vi "Global_HW_Address_Assignments.vi"() -> ()   [LabVIEW 2017]
uses:
  <vilib>/Rock Robotics/WPI/Joystick/WPI_JoystickDeviceEnum.ctl
  <vilib>/Rock Robotics/SystemInterfaces/DIO/FPGA_DIOChannel.ctl
  Claw Testing/Systems/WCDrive2018/Cluster_WCDrive_SetupData.ctl
  <vilib>/Rock Robotics/SystemInterfaces/AI/FPGA_AIChannel.ctl
  <vilib>/Rock Robotics/WPI/Solenoid/WPI_SolenoidChannel.ctl
  _SHARE ALL/RoboRio Share All/SRX Share All/TypeDefs SRX/Cluster_SRX_OPEN Data.ctl
panel:
  in  "InTake Setup":T1
  in  "WC Shift":T2
  in  "Sonar Scaling Factor":dbl=0.0235
  in  "Sonar Average Bits":u8
  in  "Sonar Channel":T3=enum."AI 3"
  in  "HW SETUP_WC Drive":T4={"Left Master"=15, "Invert Left Master"=TRUE, "Left Slave"=11, "Invert Left Slave"=FALSE, "Right Master"=16, "Invert Right Master"=TRUE, "Right Slave"=10, "Invert Right Slave"=FALSE, "Invert Left Encoder"=FALSE, "Invert Right Encoder"=FALSE}
  in  "Motor ID":u8
  in  "DIO Channel":T5=enum."DIO 1"
  in  "Button Board":T6=enum."USB 1"
  in  "Joystick":T6
  out "Invert Climber Motor":bool
  in  "Climber Motor":u8=5
  # "#HW_Adress\nAssign Motor Addresses\nWhen Given\nAssign in Global_HW_Address_Assignment.vi"
  # "#HW_Assigments These globals are used to assign\nthe HW settings for the robot. HW state machines should\nuse these global variables to ease updates if any HW\nchanges have been made."
  # "Sonar"
  # "Controllers"
  # "Climber"
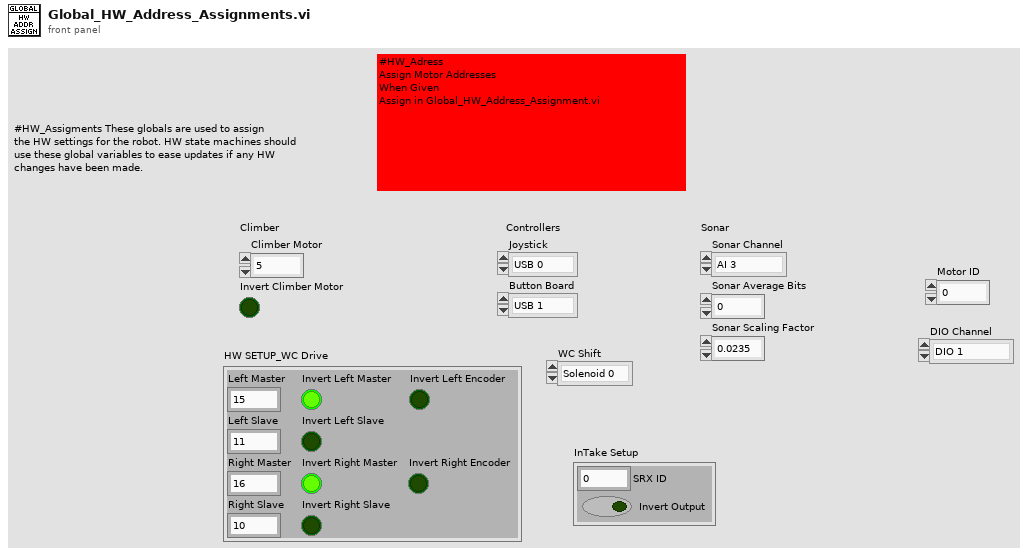
[diagram p1: front panel]
types:
  T1 = typedef "Cluster_SRX_OPEN Data.ctl" = cluster{"SRX ID":u8, "Invert Output":bool}
  T2 = typedef "WPI_SolenoidChannel.ctl" = enum8{"Solenoid 0", "Solenoid 1", "Solenoid 2", "Solenoid 3", "Solenoid 4", "Solenoid 5", "Solenoid 6", "Solenoid 7", "Invalid"}
  T3 = typedef "FPGA_AIChannel.ctl" = enum8{"AI 0", "AI 1", "AI 2", "AI 3", "AI MXP 0", "AI MXP 1", "AI MXP 2", "AI MXP 3", "Invalid"}
  T4 = typedef "Cluster_WCDrive_SetupData.ctl" = cluster{"Left Master":u8, "Invert Left Master":bool, "Left Slave":u8, "Invert Left Slave":bool, "Right Master":u8, "Invert Right Master":bool, "Right Slave":u8, "Invert Right Slave":bool, "Invert Left Encoder":bool, "Invert Right Encoder":bool}
  T5 = typedef "FPGA_DIOChannel.ctl" = enum8{"DIO 0", "DIO 1", "DIO 2", "DIO 3", "DIO 4", "DIO 5", "DIO 6", "DIO 7", "DIO 8", "DIO 9", "DIO MXP 0", "DIO MXP 1", "DIO MXP 2", "DIO MXP 3", "DIO MXP 4", "DIO MXP 5", "DIO MXP 6", "DIO MXP 7", "DIO MXP 8", "DIO MXP 9", "DIO MXP 10", "DIO MXP 11", "DIO MXP 12", "DIO MXP 13", "DIO MXP 14", "DIO MXP 15", "SPI Port CS1", "SPI Port CS2", "SPI Port CS3", "SPI Port MISO", "SPI Port MOSI", "Invalid"}
  T6 = typedef "WPI_JoystickDeviceEnum.ctl" = enum16{"USB 0", "USB 1", "USB 2", "USB 3", "USB 4", "USB 5"}
diagram:
